vi "test.recursiveFolderList.vi"() -> ()   [LabVIEW 2017]
panel:
  out "All Files in Dir 2":path[](array[path])
  out "All Files in Dir 2":path[](array[path])
  out "All Files in Dir":path[](array[path])
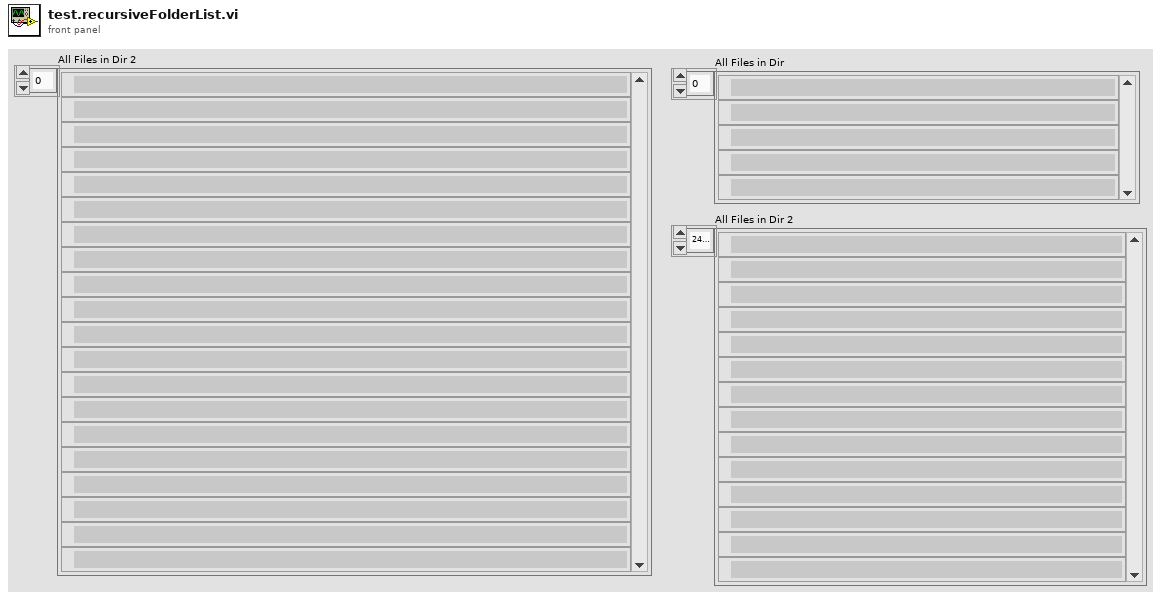
[diagram p1: front panel]
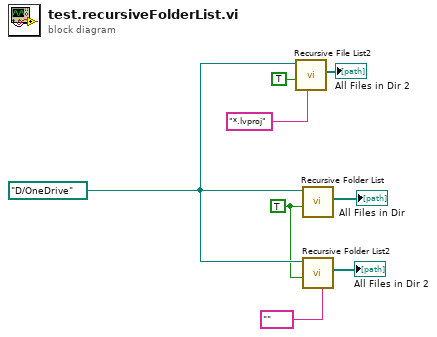
[diagram p0: block diagram]
diagram:
  w2 = TRUE ("Continue Recursing on Error? (F)")
  w8 = path "D:/OneDrive" ("Folder Path")
  n1 = call "Recursive File List2.vi"("pattern"="*.lvproj", "Continue Recursing on Error? (F)"=TRUE, "Folder Path"=w8) -> ("All Files in Dir"=→"All Files in Dir 2":path[])  [unwired: 4 in, 4 out]
  n2 = call "Recursive Folder List.vi"("Continue Recursing on Error? (F)"=w2, "Folder Path"=w8) -> ("All Folders"=→"All Files in Dir":path[])  [unwired: 6 in, 3 out]
  n3 = call "Recursive Folder List2.vi"("Folders to Exclude\nREP ( ^[_.] as Default)\nempty to disable this feature"="" ("REP ( ^[_.] as Default)\nempty to disable this feature"), "Continue Recursing on Error? (F)"=w2, "Folder Path"=w8) -> ("All Folders"=→"All Files in Dir 2":path[])  [unwired: 5 in, 3 out]
